vi "图像采集存储AVI&BMP.vi"() -> ()   [LabVIEW 2017]
uses:
  <vilib>/userdefined/High Color/IMAQdx.ctl
  <vilib>/vision/driver/NI_Vision_Acquisition_Software.lvlib
  <vilib>/vision/NI_Vision_Development_Module.lvlib
panel:
  in  "保存视频":bool
  in  "停止按钮":bool
  in  "保存图片":bool
  out "Image":T1(plugin-control)
  in  "Session In":T2="cam0"
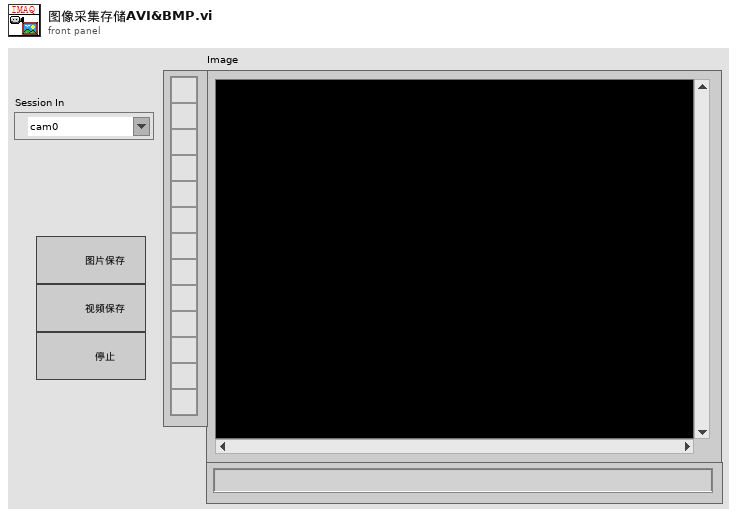
[diagram p1: front panel]
types:
  T1 = typedef "IMAQ Image.ctl" = refnum<image>
  T2 = typedef "IMAQdx.ctl" = refnum<k21>
  T3 = typedef "Image Type" = u32
  T4 = typedef "AviRefnum.ctl" = refnum<k1>
  T5 = cluster{"Desired Font (Application)":enum16{"User-specified Font", "Application Font", "System Font", "Dialog Font"}, "[User-specified Font]":cluster{"Font Name":string, "Size":i16, "Strikeout?":bool, "Italic?":bool, "Underline?":bool, "Outline?":bool, "Shadow?":bool, "Bold?":bool, "Rotation Angle":dbl}, "Horizontal Alignment":i16, "Vertical Alignment":i16}
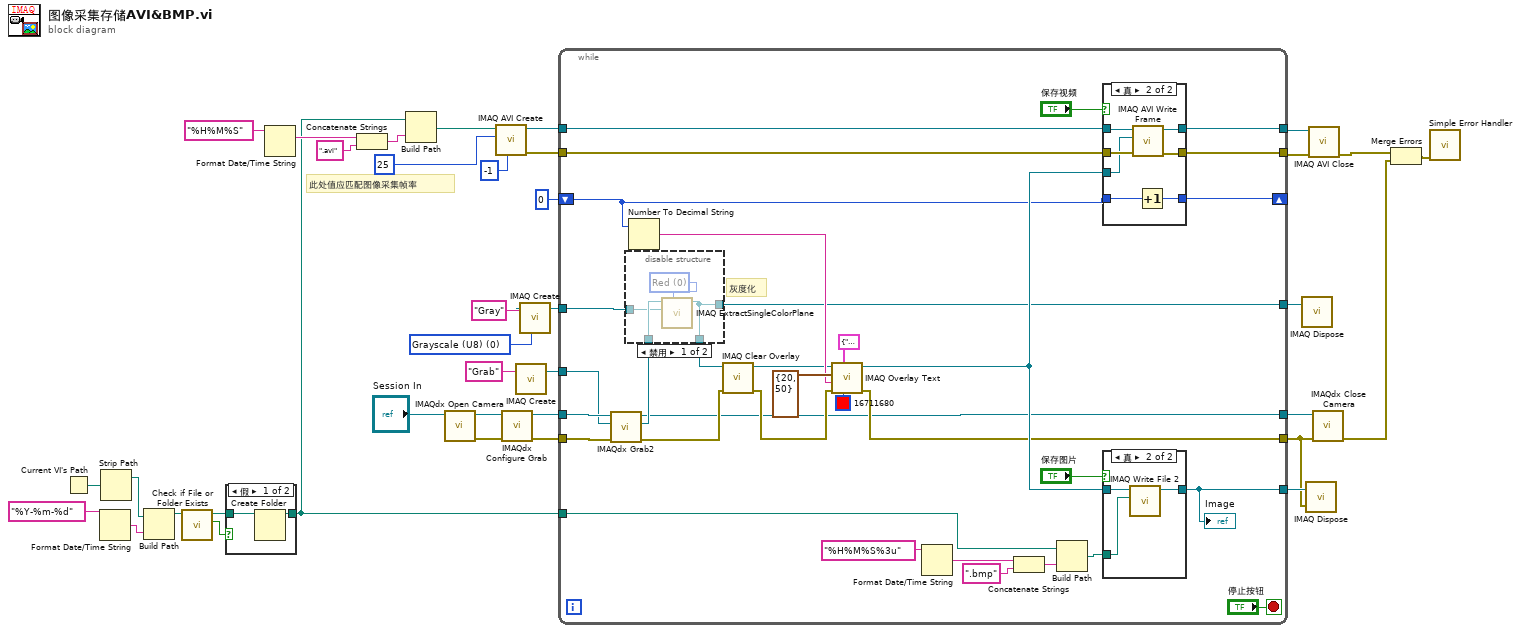
[diagram p0: block diagram]
diagram:
  w11 = T3 0 items=["Grayscale (U8)", "Grayscale (I16)", "Grayscale (SGL)", "Complex (CSG)", "RGB (U32)", "HSL (U32)", "RGB (U64)", "Grayscale (U16)"] ("Image Type")
  # "此处值应匹配图像采集帧率"
  n1 = Current VI's Path() -> (path=w4:path)
  n2 = Format Date/Time String(time format string (%c)="%Y-%m-%d" ("时间格式字符串(%c)")) -> (date/time string=w9:string)  [unwired: 2 in]
  n3 = Strip Path(path=w4) -> (stripped path=w8:path)  [unwired: 1 out]
  n4 = Build Path(base path=w8, name or relative path=w9) -> (appended path=w7:path)
  n5 = call <vilib>:"Check if File or Folder Exists.vi"("path"=w7) -> ("file or folder exists?"=w5:bool, "dup path"=w6:path)  [unwired: 8 in, 1 out]
  n6 = case shown="假" w5 {
    tunnel: w6 -> [w39 w40]
    tunnel: [w38 w40] -> w2
    frame False {
      n7 = Create Folder(path (use dialog)=w39) -> (created path=w38:path)  [unwired: 2 in, 2 out]
    }
    frame True {
    }
  }
  n8 = Format Date/Time String(time format string (%c)="%H%M%S" ("时间格式字符串(%c)")) -> (date/time string=w24:string)  [unwired: 2 in]
  n9 = Concatenate Strings(w24, ".avi" ("字符串")) -> (w26:string)
  n10 = Build Path(base path=w2, name or relative path=w26) -> (appended path=w20:path)
  n11 = call <vilib>:"IMAQdx Open Camera.vi"("Session In"="Session In") -> ("error out"=w37:errorcluster, "Session Out"=w36:T2)  [unwired: 9 in]
  n12 = call "IMAQ AVI Create"("quality"=-1 ("Quality"), "Frames Per Second"=u32 25, "AVI Path"=w20) -> ("error out"=w18:errorcluster, "Avi Refnum"=w19:T4)  [unwired: 7 in]
  n13 = call <vilib>:"IMAQdx Configure Grab.vi"("error in"=w37, "Session In"=w36) -> ("error out"=w34:errorcluster, "Session Out"=w33:T2)  [unwired: 8 in]
  n14 = call "IMAQ Create"("Image Name"="Grab") -> ("New Image"=w31:T1)  [unwired: 4 in, 1 out]
  n15 = call "IMAQ Create"("Image Name"="Gray", "Image Type"=w11) -> ("New Image"=w12:T1)  [unwired: 3 in, 1 out]
  n16 = while {
    tunnel: w34 -> [w73]
    tunnel: w33 -> [w72]
    tunnel: w31 -> [w71]
    tunnel: [w42] -> w30
    tunnel: [w56] -> w28
    tunnel: [w70] -> w29
    tunnel: [w62] -> w15
    tunnel: [w61] -> w17
    tunnel: w19 -> [w60]
    tunnel: w18 -> [w58]
    shift-right: [w52] -> _
    shift-left: 0 -> [w51]
    tunnel: w12 -> [w44]
    tunnel: [w43] -> w10
    tunnel: w2 -> [w41]
    stop <- "停止按钮" stop-if-true
    # "灰度化"
    n17 = call <vilib>:"IMAQdx Grab2.vi"("error in"=w73, "Image In"=w71, "Session In"=w72) -> ("error out"=w48:errorcluster, "Image Out"=w46:T1, "Session Out"=w42:T2)  [unwired: 5 in, 1 out]
    n18 = disable-structure shown="禁用" {
      disable-tunnel: w46 -> [w76 w79]
      disable-tunnel: [w74 w79] -> w45
      disable-tunnel: w44 -> [w75 w78]
      disable-tunnel: [w74 w78] -> w43
      frame Disabled {
        w77 = 0 items=["Red", "Green", "Blue", "Hue", "Saturation", "Luminance", "Value", "Intensity"] ("Color Plane")
        n19 = call "IMAQ ExtractSingleColorPlane"("Color Plane"=w77, "Image Dst"=w75, "Image Src"=w76) -> ("Image Dst Out"=w74:T1)  [unwired: 1 in, 7 out]
      }
      frame Enabled {
      }
    }
    n20 = Number To Decimal String(number=w51) -> (decimal integer string=w50:string)  [unwired: 1 in]
    n21 = call "IMAQ Clear Overlay"("error in (no error)"=w48, "Image"=w45) -> ("error out"=w47:errorcluster, "Image Out"=w49:T1)  [unwired: 8 in]
    n22 = call "IMAQ Overlay Text"("Text Color (black)"=u32 16711680, "Font, Size & Style"=T5 {"Desired Font (Application)"=enum."System Font", "[User-specified Font]"={"Font Name"="", "Size"=30, "Strikeout?"=FALSE, "Italic?"=FALSE, "Underline?"=FALSE, "Outline?"=FALSE, "Shadow?"=FALSE, "Bold?"=FALSE, "Rotation Angle"=0.0}, "Horizontal Alignment"=0, "Vertical Alignment"=0}, "error in (no error)"=w47, "String"=w50, "Origin"=cluster{"X":i32, "Y":i32} {"X"=20, "Y"=50}, "Image"=w49) -> ("error out"=w56:errorcluster, "Image Out"=w57:T1)  [unwired: 4 in]
    n23 = Format Date/Time String(time format string (%c)="%H%M%S%3u" ("时间格式字符串(%c)")) -> (date/time string=w64:string)  [unwired: 2 in]
    n24 = Concatenate Strings(w64, ".bmp" ("字符串")) -> (w63:string)
    n25 = Build Path(base path=w41, name or relative path=w63) -> (appended path=w69:path)
    n26 = case shown="真" "保存视频" {
      tunnel: [w82 w88] -> w62
      tunnel: [w81 w86] -> w61
      tunnel: w60 -> [w82 w89]
      tunnel: w57 -> [_ w85]
      tunnel: w58 -> [w81 w87]
      tunnel: [w80 w83] -> w52
      tunnel: w51 -> [w80 w84]
      frame False {
      }
      frame True {
        n27 = call "IMAQ AVI Write Frame"("error in (no error)"=w87, "Image"=w85, "Avi Refnum"=w89) -> ("error out"=w86:errorcluster, "Avi Refnum (duplicate)"=w88:T4)  [unwired: 7 in]
        n28 = Increment(x=w84) -> (x+1=w83:i32)
      }
    }
    n29 = case shown="真" "保存图片" {
      tunnel: w57 -> [w90 w93]
      tunnel: [w90 w92] -> w70
      tunnel: w69 -> [_ w91]
      frame False {
      }
      frame True {
        n30 = call-poly "IMAQ Write File 2"("File Path"=w91, "Image"=w93) -> ("Image Out (duplicate)"=w92:T1)  [unwired: 8 in, 1 out]
      }
    }
    "Image" <- w70
  }
  n31 = call "IMAQ Dispose"("Image"=w10) -> ()  [unwired: 5 in, 1 out]
  n32 = call "IMAQ Dispose"("Image"=w29, "error in (no error)"=w28) -> ()  [unwired: 4 in, 1 out]
  n33 = call "IMAQ AVI Close"("error in (no error)"=w17, "Avi Refnum"=w15) -> ("error out"=w16:errorcluster)  [unwired: 9 in]
  n34 = call <vilib>:"IMAQdx Close Camera.vi"("error in"=w28, "Session In"=w30) -> ("error out"=w27:errorcluster)  [unwired: 9 in]
  n35 = Merge Errors(w16, w27) -> (w1:errorcluster)
  n36 = call <vilib>:"Simple Error Handler.vi"("error in (no error)"=w1) -> ()  [unwired: 4 in, 5 out]
